vi "Configure Ossiloscope Settings.vi"(8 "error in":errorcluster, 10 "input settings":T1={"LeCroy IP"="169.254.20.90", "Ch1"={"On/Off"=FALSE, "Bandwidth (Dropdown)"=0, "Vertical Range (V)"=5000.0, "Vertical Offset (V)"=0.0}, "Ch2"={"On/Off"=FALSE, "Bandwidth (Dropdown)"=0, "Vertical Range (V)"=0.2, "Vertical Offset (V)"=0.0}, "Ch3"={"On/Off"=TRUE, "Bandwidth (Dropdown)"=0, "Vertical Range (V)"=1.2, "Vertical Offset (V)"=0.0}, "Ch4"={"On/Off"=TRUE, "Bandwidth (Dropdown)"=0, "Vertical Range (V)"=0.2, "Vertical Offset (V)"=0.0}, "T axis"={"Time base (s/div)"=0.0002, "Time offset (s)"=0.0, "Max Sample Points"=0}, "Trig"={"Trigger mode"=2, "Trigger Slope"=0, "Trigger Source"=1, "Trigger Level (V)"=0.04}, "Timeout (ms)"=0.0} caption="Settings" {"Trig"."Trigger mode" items=["Auto", "Normal", "Single", "Single, auto trigger"]; "Trig"."Trigger Slope" items=["Rising", "Falling"]; "Trig"."Trigger Source" items=["Channel 1", "Channel 2", "Channel 3", "Channel 4", "External", "Power Line"]; "Trig"."Trigger Level (V)" format="%#_6p"; "T axis"."Max Sample Points" format="%.0p" items=["50"=50, "100"=100, "250"=250, "500"=500, "1000"=1000, "2500"=2500, "5K"=5000, "10K"=10000, "25K"=25000, "50K"=50000, "100K"=100000, "250K"=250000, "500K"=500000, "1M"=1000000, "2M"=2000000, "2.5M"=2500000, "5M"=5000000, "10M"=10000000, "25M"=25000000, "50M"=50000000, "100M"=100000000]; "T axis"."Time base (s/div)" format="%#_6p"; "Ch4"."Bandwidth (Dropdown)" items=["Full", "20MHZ", "25MHZ", "200MHZ", "250MHZ", "1GHZ", "3GHZ", "4GHZ"]; "Ch3"."Bandwidth (Dropdown)" items=["Full", "20MHZ", "25MHZ", "200MHZ", "250MHZ", "1GHZ", "3GHZ", "4GHZ"]; "Ch2"."Bandwidth (Dropdown)" items=["Full", "20MHZ", "25MHZ", "200MHZ", "250MHZ", "1GHZ", "3GHZ", "4GHZ"]; "Ch1"."Bandwidth (Dropdown)" items=["Full", "20MHZ", "25MHZ", "200MHZ", "250MHZ", "1GHZ", "3GHZ", "4GHZ"]}, 11 "VISA resource name in":refnum<visa-resource-name>) -> (0 "error out":errorcluster, 1 "Channels to read out":i32[](array[numeric]), 2 "output settings":T1={"LeCroy IP"="169.254.20.90", "Ch1"={"On/Off"=FALSE, "Bandwidth (Dropdown)"=0, "Vertical Range (V)"=5000.0, "Vertical Offset (V)"=0.0}, "Ch2"={"On/Off"=FALSE, "Bandwidth (Dropdown)"=0, "Vertical Range (V)"=0.2, "Vertical Offset (V)"=0.0}, "Ch3"={"On/Off"=TRUE, "Bandwidth (Dropdown)"=0, "Vertical Range (V)"=1.2, "Vertical Offset (V)"=0.0}, "Ch4"={"On/Off"=TRUE, "Bandwidth (Dropdown)"=0, "Vertical Range (V)"=0.2, "Vertical Offset (V)"=0.0}, "T axis"={"Time base (s/div)"=0.0002, "Time offset (s)"=0.0, "Max Sample Points"=0}, "Trig"={"Trigger mode"=2, "Trigger Slope"=0, "Trigger Source"=1, "Trigger Level (V)"=0.04}, "Timeout (ms)"=0.0} caption="Settings" {"Trig"."Trigger mode" items=["Auto", "Normal", "Single", "Single, auto trigger"]; "Trig"."Trigger Slope" items=["Rising", "Falling"]; "Trig"."Trigger Source" items=["Channel 1", "Channel 2", "Channel 3", "Channel 4", "External", "Power Line"]; "Trig"."Trigger Level (V)" format="%#_6p"; "T axis"."Max Sample Points" format="%.0p" items=["50"=50, "100"=100, "250"=250, "500"=500, "1000"=1000, "2500"=2500, "5K"=5000, "10K"=10000, "25K"=25000, "50K"=50000, "100K"=100000, "250K"=250000, "500K"=500000, "1M"=1000000, "2M"=2000000, "2.5M"=2500000, "5M"=5000000, "10M"=10000000, "25M"=25000000, "50M"=50000000, "100M"=100000000]; "T axis"."Time base (s/div)" format="%#_6p"; "Ch4"."Bandwidth (Dropdown)" items=["Full", "20MHZ", "25MHZ", "200MHZ", "250MHZ", "1GHZ", "3GHZ", "4GHZ"]; "Ch3"."Bandwidth (Dropdown)" items=["Full", "20MHZ", "25MHZ", "200MHZ", "250MHZ", "1GHZ", "3GHZ", "4GHZ"]; "Ch2"."Bandwidth (Dropdown)" items=["Full", "20MHZ", "25MHZ", "200MHZ", "250MHZ", "1GHZ", "3GHZ", "4GHZ"]; "Ch1"."Bandwidth (Dropdown)" items=["Full", "20MHZ", "25MHZ", "200MHZ", "250MHZ", "1GHZ", "3GHZ", "4GHZ"]}, 3 "VISA resource name out":refnum<visa-resource-name>)   [LabVIEW 2013]
uses:
  Settings_TypeDef.ctl
  <instrlib>/LeCroy Wave Series/Public/Configure/Configure Edge Trigger.vi
  <instrlib>/LeCroy Wave Series/LeCroy Wave Series.lvlib
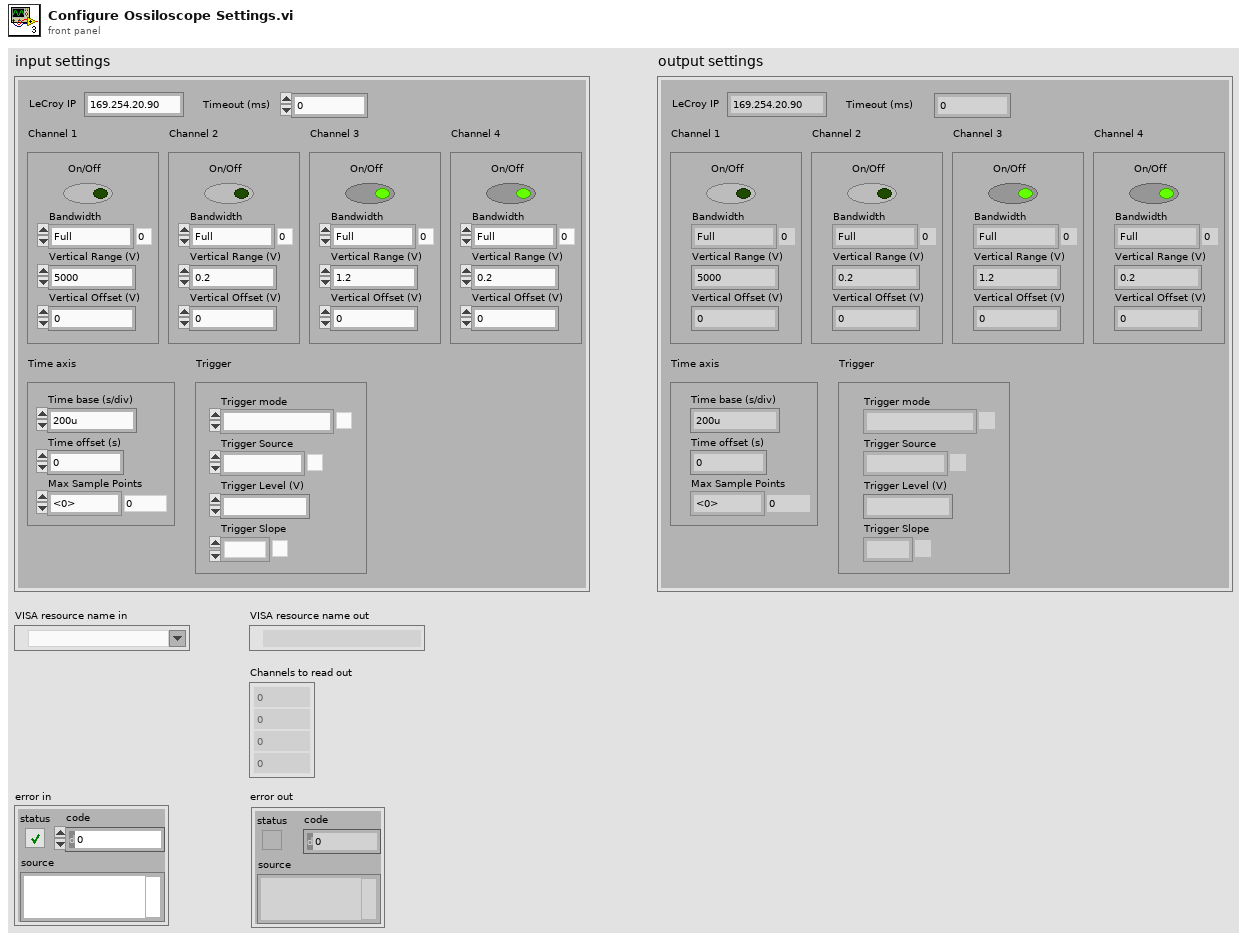
[diagram p1: front panel]
types:
  T1 = typedef "Settings_TypeDef.ctl" = cluster{"LeCroy IP":string, "Ch1":cluster{"On/Off":bool, "Bandwidth (Dropdown)":u16, "Vertical Range (V)":dbl, "Vertical Offset (V)":dbl}, "Ch2":cluster{"On/Off":bool, "Bandwidth (Dropdown)":u16, "Vertical Range (V)":dbl, "Vertical Offset (V)":dbl}, "Ch3":cluster{"On/Off":bool, "Bandwidth (Dropdown)":u16, "Vertical Range (V)":dbl, "Vertical Offset (V)":dbl}, "Ch4":cluster{"On/Off":bool, "Bandwidth (Dropdown)":u16, "Vertical Range (V)":dbl, "Vertical Offset (V)":dbl}, "T axis":cluster{"Time base (s/div)":dbl, "Time offset (s)":dbl, "Max Sample Points":i32}, "Trig":cluster{"Trigger mode":u16, "Trigger Slope":u16, "Trigger Source":u16, "Trigger Level (V)":dbl}, "Timeout (ms)":dbl}
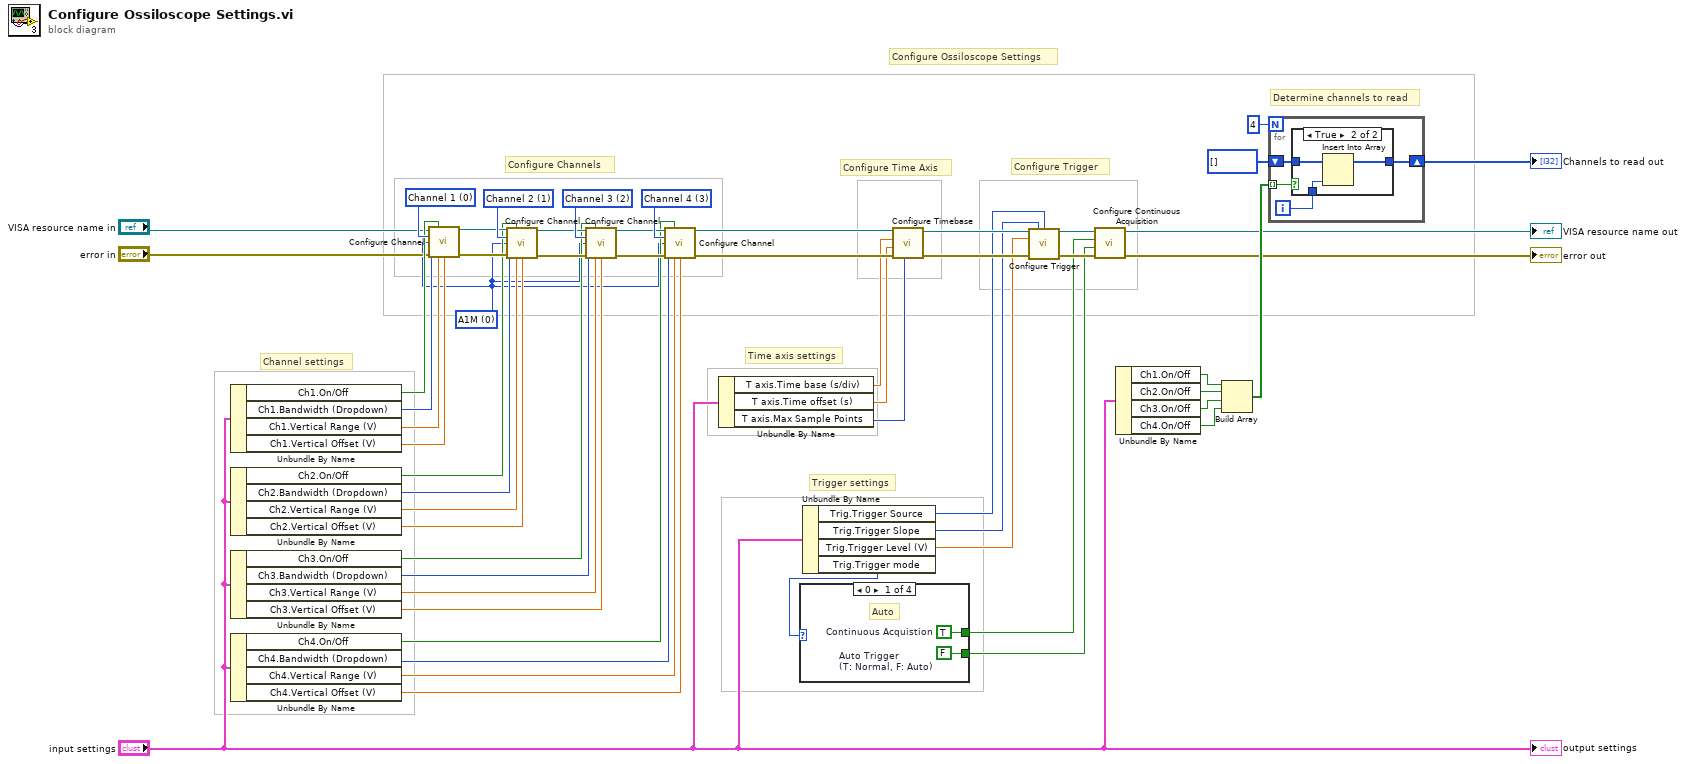
[diagram p0: block diagram]
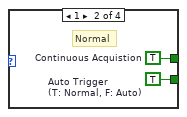
[diagram p3: hidden frame]
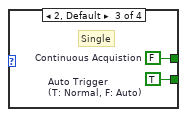
[diagram p4: hidden frame]
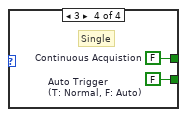
[diagram p5: hidden frame]
diagram:
  w1 = u16 0 items=["A1M", "D1M", "D50", "Ground", "DC", "AC"] ("Vertical Coupling (0: A1M)")
  w52 = u16 3 items=["Channel 1", "Channel 2", "Channel 3", "Channel 4"] ("Source (0: Channel 1)")
  w53 = u16 2 items=["Channel 1", "Channel 2", "Channel 3", "Channel 4"] ("Source (0: Channel 1)")
  w54 = u16 1 items=["Channel 1", "Channel 2", "Channel 3", "Channel 4"] ("Source (0: Channel 1)")
  w55 = u16 0 items=["Channel 1", "Channel 2", "Channel 3", "Channel 4"] ("Source (0: Channel 1)")
  # "Determine channels to read"
  # "Trigger settings"
  # "Configure Trigger"
  # "Configure Time Axis"
  # "Time axis settings"
  # "Channel settings"
  # "Configure Channels"
  # "Configure Ossiloscope Settings"
  n1 = Unbundle By Name("input settings") -> ("Ch1.On/Off"=w33:bool, "Ch1.Bandwidth (Dropdown)"=w38:u16, "Ch1.Vertical Range (V)"=w39:dbl, "Ch1.Vertical Offset (V)"=w40:dbl)
  n2 = Unbundle By Name("input settings") -> ("Ch2.On/Off"=w30:bool, "Ch2.Bandwidth (Dropdown)"=w31:u16, "Ch2.Vertical Range (V)"=w32:dbl, "Ch2.Vertical Offset (V)"=w29:dbl)
  n3 = Unbundle By Name("input settings") -> ("Ch3.On/Off"=w24:bool, "Ch3.Bandwidth (Dropdown)"=w23:u16, "Ch3.Vertical Range (V)"=w22:dbl, "Ch3.Vertical Offset (V)"=w21:dbl)
  n4 = Unbundle By Name("input settings") -> ("Ch4.On/Off"=w26:bool, "Ch4.Bandwidth (Dropdown)"=w27:u16, "Ch4.Vertical Range (V)"=w28:dbl, "Ch4.Vertical Offset (V)"=w25:dbl)
  n5 = call <instrlib>:"Configure Channel.vi"("VISA resource name"="VISA resource name in", "Enable Channel (T:On)"=w33, "Bandwidth (0: Full)"=w38, "Channel (0: Channel 1)"=w55, "Vertical Coupling (0: A1M)"=w1, "error in (no error)"="error in", "Vertical Range (10.0 V)"=w39, "Vertical Offset (0.0 V)"=w40) -> ("VISA resource name out"=w51:refnum<visa-resource-name>, "error out"=w50:errorcluster)  [unwired: 6 in]
  n6 = call <instrlib>:"Configure Channel.vi"("VISA resource name"=w51, "Enable Channel (T:On)"=w30, "Bandwidth (0: Full)"=w31, "Channel (0: Channel 1)"=w54, "Vertical Coupling (0: A1M)"=w1, "error in (no error)"=w50, "Vertical Range (10.0 V)"=w32, "Vertical Offset (0.0 V)"=w29) -> ("VISA resource name out"=w48:refnum<visa-resource-name>, "error out"=w49:errorcluster)  [unwired: 6 in]
  n7 = call <instrlib>:"Configure Channel.vi"("VISA resource name"=w48, "Enable Channel (T:On)"=w24, "Bandwidth (0: Full)"=w23, "Channel (0: Channel 1)"=w53, "Vertical Coupling (0: A1M)"=w1, "error in (no error)"=w49, "Vertical Range (10.0 V)"=w22, "Vertical Offset (0.0 V)"=w21) -> ("VISA resource name out"=w47:refnum<visa-resource-name>, "error out"=w46:errorcluster)  [unwired: 6 in]
  n8 = call <instrlib>:"Configure Channel.vi"("VISA resource name"=w47, "Enable Channel (T:On)"=w26, "Bandwidth (0: Full)"=w27, "Channel (0: Channel 1)"=w52, "Vertical Coupling (0: A1M)"=w1, "error in (no error)"=w46, "Vertical Range (10.0 V)"=w28, "Vertical Offset (0.0 V)"=w25) -> ("VISA resource name out"=w45:refnum<visa-resource-name>, "error out"=w44:errorcluster)  [unwired: 6 in]
  n9 = Unbundle By Name("input settings") -> ("T axis.Time base (s/div)"=w20:dbl, "T axis.Time offset (s)"=w19:dbl, "T axis.Max Sample Points"=w18:i32)
  n10 = Unbundle By Name("input settings") -> ("Trig.Trigger Source"=w11:u16, "Trig.Trigger Slope"=w10:u16, "Trig.Trigger Level (V)"=w9:dbl, "Trig.Trigger mode"=w8:u16)
  n11 = case shown="0" w8 {
    tunnel: [w57 w59 w61 w63] -> w12
    tunnel: [w56 w58 w60 w62] -> w13
    frame 0 {
      w56 = FALSE  # Auto Trigger (T: Normal, F: Auto)
      w57 = TRUE  # Continuous Acquistion
      # "Auto"
    }
    frame 1 {
      w58 = TRUE  # Auto Trigger (T: Normal, F: Auto)
      w59 = TRUE  # Continuous Acquistion
      # "Normal"
    }
    frame 2, Default {
      w60 = TRUE  # Auto Trigger (T: Normal, F: Auto)
      w61 = FALSE  # Continuous Acquistion
      # "Single"
    }
    frame 3 {
      w62 = FALSE  # Auto Trigger (T: Normal, F: Auto)
      w63 = FALSE  # Continuous Acquistion
      # "Single"
    }
  }
  n12 = call <instrlib>:"Configure Timebase.vi"("Maximum Sample Points (500)"=w18, "error in (no error)"=w44, "Position (0.0 s)"=w19, "Timebase (0.0005 s)"=w20, "VISA resource name"=w45) -> ("error out"=w14:errorcluster, "VISA resource name out"=w17:refnum<visa-resource-name>)  [unwired: 5 in]
  n13 = call-poly <instrlib>:"Configure Trigger.vi"("VISA resource name"=w17, "Trigger Slope (0: Rising)"=w10, "Trigger Source (0: Channel 1)"=w11, "Trigger Level (0.0 V)"=w9, "error in (no error)"=w14) -> ("VISA resource name out"=w16:refnum<visa-resource-name>, "error out"=w15:errorcluster)  [unwired: 9 in]
  n14 = call <instrlib>:"Configure Continuous Acquisition.vi"("error in (no error)"=w15, "Auto Trigger Enabled (T: Normal)"=w13, "Continuous Acquisition Mode (T: On)"=w12, "VISA resource name"=w16) -> ("error out"=→"error out":errorcluster, "VISA resource name out"=→"VISA resource name out":refnum<visa-resource-name>)  [unwired: 6 in]
  n15 = Unbundle By Name("input settings") -> ("Ch1.On/Off"=w37:bool, "Ch2.On/Off"=w36:bool, "Ch3.On/Off"=w35:bool, "Ch4.On/Off"=w34:bool)
  n16 = Build Array(w37, w36, w35, w34) -> (w43:bool[])
  n17 = for {
    N: 4 -> [_]
    tunnel: w43 -> [w64] mode=indexing
    shift-right: [w65] -> w2
    shift-left: i32[] [] -> [w66]
    i -> [w67]
    n18 = case shown="True" w64 {
      tunnel: w67 -> [_ w71]
      tunnel: w66 -> [w68 w70]
      tunnel: [w68 w69] -> w65
      frame False {
      }
      frame True {
        n19 = Insert Into Array(array=w70, new element=w71) -> (w69:i32[])  [unwired: 1 in]
      }
    }
  }
  "Channels to read out" <- w2
  "output settings" <- "input settings"
